vi "S2C_Access_CreateDSN.vi"(8 "Error In":errorcluster, 11 "Path In":path) -> (0 "Error Out":errorcluster, 3 "Path Out":path)   [LabVIEW 2015]
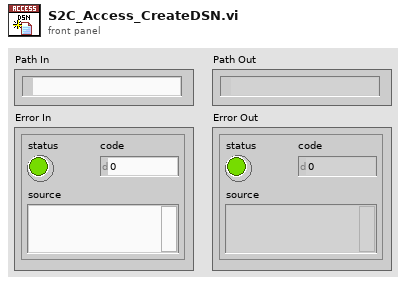
[diagram p1: front panel]
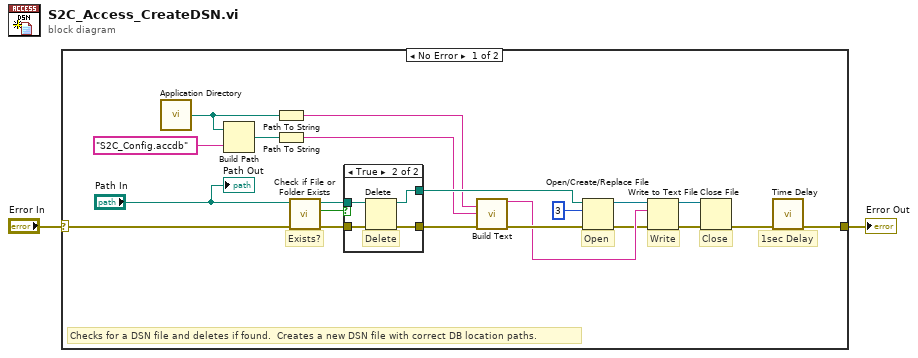
[diagram p0: block diagram]
diagram:
  n1 = case shown="No Error" "Error In" {
    selector: "Error In" -> [w6 w30]
    tunnel: [w3 w30] -> w1
    frame No Error {
      # "1sec Delay"
      # "Exists?"
      # "Checks for a DSN file and deletes if found.  Creates a new DSN file with correct DB location paths."
      # "Close"
      # "Write"
      # "Open"
      n2 = call <vilib>:"Application Directory.vi"() -> ("Application Directory"=w14:path)
      n3 = Build Path(base path=w14, name or relative path="S2C_Config.accdb") -> (appended path=w12:path)
      n4 = Path To String(path=w14) -> (string=w13:string)
      n5 = Path To String(path=w12) -> (string=w11:string)
      n6 = call <vilib>:"Check if File or Folder Exists.vi"("error in (no error)"=w6, "path"="Path In") -> ("error out"=w20:errorcluster, "file or folder exists?"=w19:bool, "dup path"=w18:path)  [unwired: 7 in]
      n7 = case shown="True" w19 {
        tunnel: w20 -> [w24 w29]
        tunnel: w18 -> [w25 w28]
        tunnel: [w24 w27] -> w15
        tunnel: [w25 w26] -> w17
        frame False {
        }
        frame True {
          # "Delete"
          n8 = Delete(path (use dialog)=w28, error in=w29) -> (deleted path=w26:path, error out=w27:errorcluster)  [unwired: 3 in, 1 out]
        }
      }
      n9 = call "Build Text"("Dir"=w13, "File"=w11, "error in (no error)"=w15) -> ("Result"=w9:string, "error out"=w10:errorcluster)  [unwired: 11 in]
      n10 = Open/Create/Replace File(file path (use dialog)=w17, error in=w10, operation (0:open)=u16 3) -> (refnum out=w7:refnum<file>, error out=w8:errorcluster)  [unwired: 3 in, 1 out]
      n11 = Write to Text File(file (use dialog)=w7, text=w9, error in=w8) -> (refnum out=w21:refnum<file>, error out=w22:errorcluster)  [unwired: 1 in, 1 out]
      n12 = Close File(refnum=w21, error in=w22) -> (error out=w4:errorcluster)  [unwired: 1 out]
      n13 = call "Time Delay"("error in (no error)"=w4) -> ("error out"=w3:errorcluster)  [unwired: 10 in]
      "Path Out" <- "Path In"
    }
    frame Error {
    }
  }
  "Error Out" <- w1
